vi "Check for extension.vi"(8 "error in (no error)":errorcluster, 9 "extension version":string="1", 10 "extension name":string, 11 "session in":refnum<class "Session.lvclass">) -> (0 "error out":errorcluster)   [LabVIEW 2020, in "NI_SFTP.lvlib" / "Session.lvclass"]
uses:
  <vilib>/net/SFTP/Session/Session.lvclass
  <vilib>/net/SFTP/Session/Session.lvclass/Session.ctl
  <vilib>/net/SFTP/Low Level Connection/Low Level Connection.lvclass/Low Level Connection.ctl
  <vilib>/net/SFTP/Low Level Connection/Extension Pair.ctl
  <vilib>/Utility/error.llb/Error Cluster From Error Code.vi
  <vilib>/ErrorRing/Error Ring.xnode
  <vilib>/net/SSH/NI_SSH.lvlib
  <vilib>/net/SFTP/Low Level Connection/Low Level Connection.lvclass
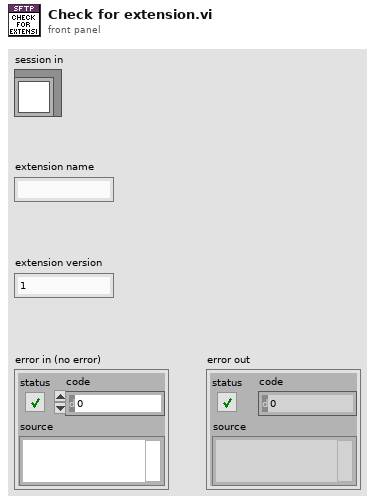
[diagram p1: front panel]
types:
  T1 = typedef "NI_SFTP.lvlib/Low Level Connection.lvclass/Extension Pair.ctl" = cluster{"name":string, "version":string}
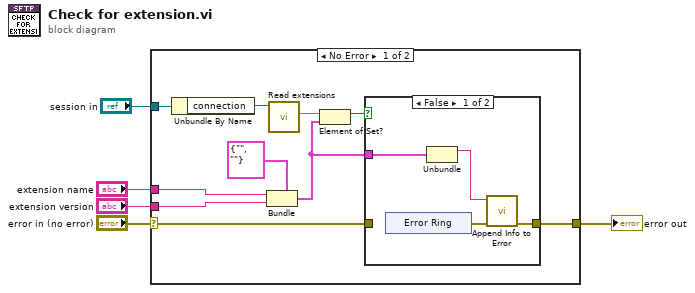
[diagram p0: block diagram]
diagram:
  n1 = case shown="No Error" "error in (no error)" {
    selector: "error in (no error)" -> [w12 w25]
    tunnel: [w13 w25] -> w5
    tunnel: "extension name" -> [w11 _]
    tunnel: "extension version" -> [w10 _]
    tunnel: "session in" -> [w7 _]
    frame No Error {
      n2 = Unbundle By Name(w7) -> ("connection"=w6:refnum<class "Low Level Connection.lvclass">)
      n3 = Bundle(cluster=T1 {"name"="", "version"=""} ("extension-pair"), "name"=w11, "version"=w10) -> (w8:T1)
      n4 = call <vilib>:"Read extensions.vi"("connection in"=w6) -> ("extensions"=w15:set{T1})  [unwired: 9 in, 1 out]
      n5 = Element of Set?(10:w8, 11:w15) -> (3:w14:bool)
      n6 = case shown="False" w14 {
        tunnel: [w16 w24] -> w13
        tunnel: w12 -> [_ w24]
        tunnel: w8 -> [w18 _]
        frame False {
          n7 = xnode "Error Ring"() -> ("error out"=w17:errorcluster)
          n8 = Unbundle(w18) -> ("name"=w19:string)  [unwired: 1 out]
          n9 = call <vilib>:"Append Info to Error.vi"("error in (no error)"=w17, "additional info"=w19) -> ("error out"=w16:errorcluster)  [unwired: 9 in]
        }
        frame True {
        }
      }
    }
    frame Error {
    }
  }
  "error out" <- w5
